vi "Close.vi"(8 "error in (no error)":errorcluster caption="错误输入（无错误）", 11 "DMM 输入":refnum<class "Keithley 2000.lvclass">) -> (0 "error out":errorcluster caption="错误输出", 3 "DMM 输出":refnum<class "Keithley 2000.lvclass">)   [LabVIEW 2020, in "DMM.lvlib" / "Keithley 2000.lvclass"]
uses:
  Keithley 2000.lvclass
  D:/Workspace/LabVIEW/LVDevClass/DMM/root/root.lvclass
  Keithley 2000.lvclass/Keithley 2000.ctl
  <instrlib>/Keithley 2000/Keithley 2000.lvlib
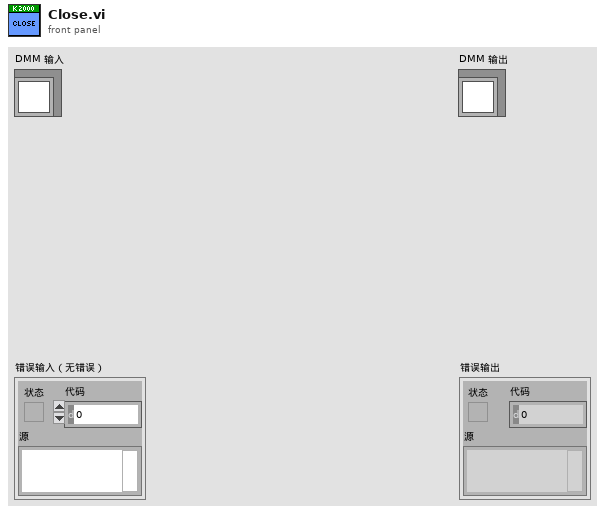
[diagram p1: front panel]
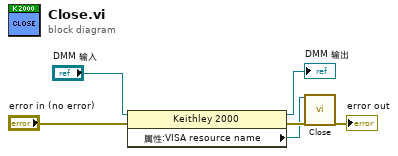
[diagram p0: block diagram]
diagram:
  n1 = property class="Keithley 2000"(reference="DMM 输入", error in="error in (no error)") -> (reference out=→"DMM 输出":refnum<class "Keithley 2000.lvclass">, error out=w5:errorcluster, "属性:VISA resource name"=w1:refnum<visa-resource-name>)
  n2 = call <instrlib>:"Close.vi"("VISA resource name"=w1, "error in (no error)"=w5) -> ("error out"=→"error out":errorcluster)  [unwired: 17 in]
